vi "Current Sense State to Word.vi"(11 "Wheel Speed Sensor State":T1) -> (3 "Current Sense Word":u16 format="%b")   [LabVIEW 2014, in "SLSC configuration Shared.lvlib"]
doc: "Converts four faults to a fault word."
uses:
  SLSC configuration Shared.lvlib
  Current Sense Calibration State.ctl
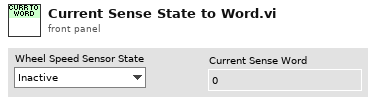
[diagram p1: front panel]
types:
  T1 = typedef "SLSC configuration Shared.lvlib/Current Sense Calibration State.ctl" = enum16{"Inactive", "Channel 1", "Channel 2", "Channel 3", "Channel 4", "Channel 5", "Channel 6", "Channel 7", "Channel 8", "Channel 9", "Channel 10", "Channel 11", "Channel 12", "Channel 13", "Channel 14", "Channel 15", "Channel 16"}
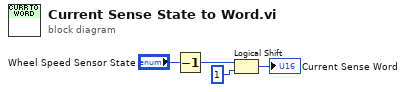
[diagram p0: block diagram]
diagram:
  n1 = Decrement(x="Wheel Speed Sensor State") -> (x-1=w2:T1)
  n2 = Logical Shift(y=w2, x=u16 1 ("y")) -> (x << y=→"Current Sense Word":u16)
